vi "Create Library For Destination.vi"(8 "error in (no error)":errorcluster, 9 "New project library name":string, 10 "Destination label":string, 11 "PPL in":refnum<class "NI_AB_API_PPL.lvclass">) -> (0 "error out":errorcluster, 3 "PPL out":refnum<class "NI_AB_API_PPL.lvclass">)   [LabVIEW 2020, in "NI_AB_API_PPL.lvclass"]
uses:
  <vilib>/AppBuilder/AB_API/PPL/NI_AB_API_PPL.lvclass
  <vilib>/AppBuilder/AB_API/common/AB_API Default Destinations.ctl
  <vilib>/AppBuilder/AB_API/Targetfile/NI_AB_API_Targetfile.lvclass
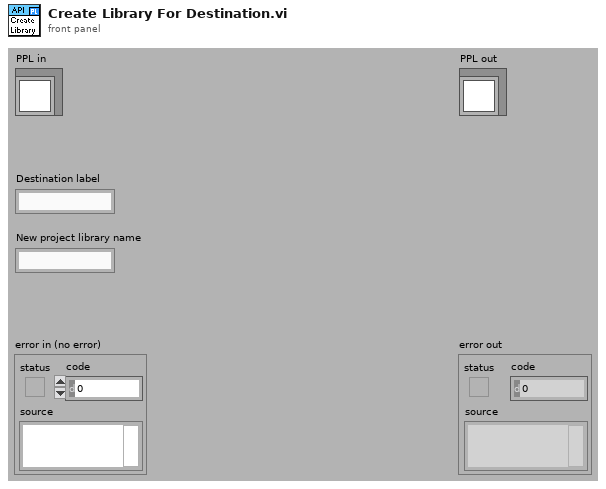
[diagram p1: front panel]
types:
  T1 = typedef "AB_API Default Destinations.ctl" = enum16{"Destination Directory", "Support Directory"}
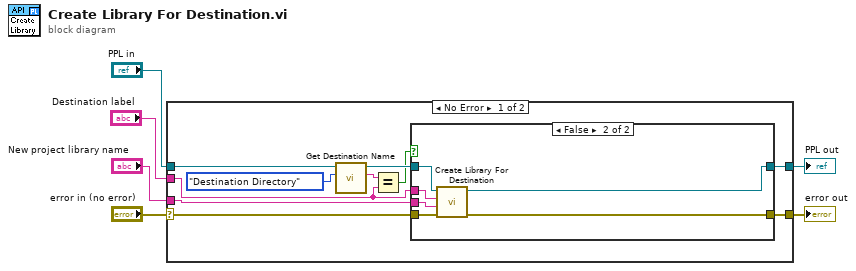
[diagram p0: block diagram]
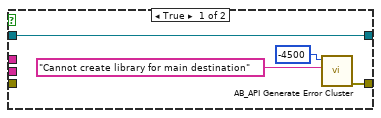
[diagram p2: hidden frame]
diagram:
  n1 = case shown="No Error" "error in (no error)" {
    selector: "error in (no error)" -> [w16 w28]
    tunnel: [w15 w28] -> w5
    tunnel: [w13 w27] -> w3
    tunnel: "PPL in" -> [w12 w27]
    tunnel: "New project library name" -> [w14 _]
    tunnel: "Destination label" -> [w8 _]
    frame No Error {
      n2 = call-dynamic "Get Destination Name.vi"("Default Destinations"=AB_API_Default_Destinations."Destination Directory", "PPL in"=w12) -> ("Destination Name"=w9:string, "PPL out"=w11:refnum<class "NI_AB_API_PPL.lvclass">)  [unwired: 7 in, 1 out]
      n3 = Equal?(x=w9, y=w8) -> (x = y?=w7:bool)
      n4 = case shown="False" w7 {
        tunnel: w16 -> [_ w23]
        tunnel: [w17 w24] -> w15
        tunnel: w14 -> [_ w22]
        tunnel: [w20 w25] -> w13
        tunnel: w11 -> [w20 w26]
        tunnel: w8 -> [_ w21]
        frame True {
          n5 = call <vilib>:"AB_API Generate Error Cluster.vi"("Additional Message"="Cannot create library for main destination", "Code"=-4500) -> ("error out"=w17:errorcluster)  [unwired: 9 in]
        }
        frame False {
          n6 = call-parent "Create Library For Destination.vi"("error in (no error)"=w23, "New project library name"=w22, "Destination label"=w21, "Build in"=w26) -> ("error out"=w24:errorcluster, "Build out"=w25:refnum<class "NI_AB_API_PPL.lvclass">)  [unwired: 6 in]
        }
      }
    }
    frame Error {
    }
  }
  "error out" <- w5
  "PPL out" <- w3
